vi "Init SPI CS Pin.vi"(4 "CS Active Low (T)":bool=TRUE, 5 "CS GPIO":i32=5, 8 "error in (no error)":errorcluster, 11 "VISA resource name in":refnum<visa-resource-name>) -> (0 "error out":errorcluster, 3 "VISA resource name":refnum<visa-resource-name>)   [LabVIEW 2023, in "CTI-Visa.lvlib"]
uses:
  Digital Direction.ctl
  CTI-Visa.lvlib
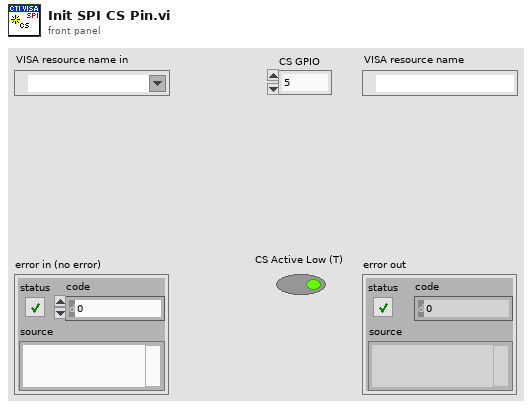
[diagram p1: front panel]
types:
  T1 = typedef "CTI-Visa.lvlib/Digital Direction.ctl" = enum16{"In", "Out"}
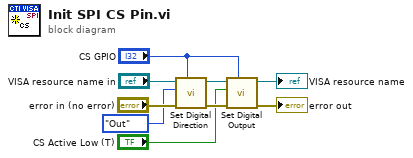
[diagram p0: block diagram]
diagram:
  n1 = call "Set Digital Direction.vi"("GPIO"="CS GPIO", "error in (no error)"="error in (no error)", "Direction"=Digital_Direction."Out", "VISA resource name in"="VISA resource name in") -> ("error out"=w5:errorcluster, "VISA resource name"=w6:refnum<visa-resource-name>)  [unwired: 6 in]
  n2 = call "Set Digital Output.vi"("GPIO"="CS GPIO", "error in (no error)"=w5, "Value"="CS Active Low (T)", "VISA resource name in"=w6) -> ("error out"=→"error out":errorcluster, "VISA resource name"=→"VISA resource name":refnum<visa-resource-name>)  [unwired: 6 in]
